vi "Sample Request Control.vi"(0 "Sample Request":bool, 2 "DOUTs OFF":bool, 4 "SimDINs":bool[](array[boolean])=[FALSE, FALSE, FALSE, FALSE, FALSE], 5 "ErrIn":errorcluster, 6 "PC ID":i32=1, 7 "SimOn":bool, 8 "PC1 In Inv":bool[](array[boolean])=[FALSE, FALSE, FALSE, FALSE, FALSE], 9 "Init":bool, 10 "Lockout Inv":bool, 11 "Reset":bool, 13 "Stop":bool) -> (14 "Request Granted":bool, 15 "Lockout Status":bool, 16 "Reset Done":bool, 17 "State":T1(ring), 18 "Busy Status":bool[](array[boolean]), 19 "ErrOut":errorcluster)   [LabVIEW 2013]
uses:
  <vilib>/DAQmx/write.llb/DAQmx Write (Digital Bool 1Line 1Point).vi
  <vilib>/DAQmx/read.llb/DAQmx Read (Digital 1D Bool NChan 1Samp 1Line).vi
  <vilib>/DAQmx/miscellaneous.llb/DAQmx Fill In Error Info.vi
  <vilib>/DAQmx/create/channels.llb/DAQmx Create Channel (DI-Digital Input).vi
  <vilib>/DAQmx/create/channels.llb/DAQmx Create Channel (DO-Digital Output).vi
panel:
  in  "PC1 In Line Grouping":i32(ring) items=["one channel for each line", "one channel for all lines"]
  in  "PC1 In Chls":tag="Dev1/port2/line0:1"
  in  "PC1 Out Line Grouping":i32(ring) items=["one channel for each line", "one channel for all lines"]
  in  "PC1 Out Chls":tag="Dev1/port1/line6"
  # "Input Parameters"
  # "ER2007"
  # "Output Parameters"
  # "Expected \"Sample Request\" Button Behavior:\n(1) A transition from FALSE to TRUE signals the start of a new\n     request.  If the other PC is not in the middle of a sample,\n     this vi sets \"Request Granted\" to TRUE and asserts the\n     \"Lockout\" line.  On the next loop iteration, \"Sample Request\"\n     must be FALSE because global 'GCD Busy' is now TRUE.\n     This vi proceeds thru if phases and returns to the 'Idle' state,\n(2)  If the other PC was processing a sample (busy), then this vi\n      proceeds to the 'Check Again x' state.  So long as the \"Sample\n      Request\" remains TRUE, the Busy line is checked every loop\n      iteration until it is either FALSE or until the \"Reset\" button is\n      pushed.  If the Busy goes FALSE, the \"Request Granted\" and\n      the \"Lockout\" lines are asserted.\n(3)  An external \"Reset\" is required to return the \"Lockout\" line to\n      FALSE.  Output Boolean \"Lockout Done\" is pulsed high and\n      can be used to reset the Global variable used for resets.\n(4) The \"Request Granted\" Boolean is pulsed TRUE for one loop\n      iteration."
  # "PC #1 Input Channels"
  # "PC #1 Output Channel"
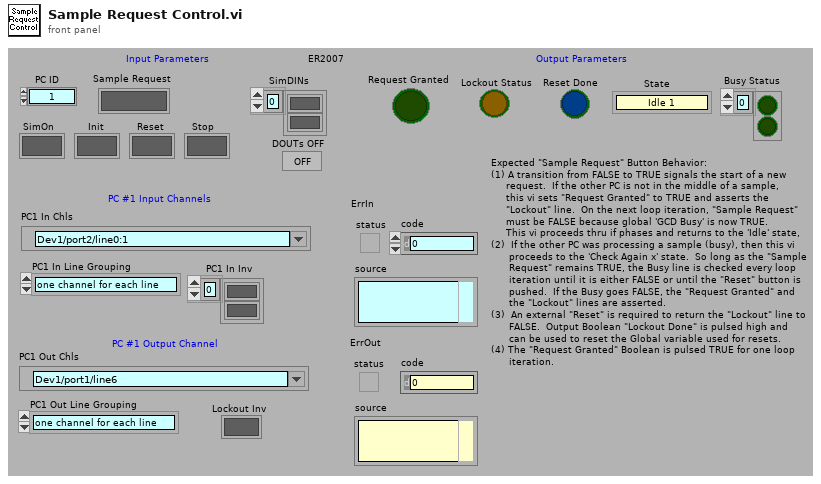
[diagram p1: front panel]
types:
  T1 = enum16{"Idle 1", "Request 1", "Check Again 1", "Done 1", "Idle 2", "Request 2", "Wait 2", "Check Again 2", "Done 2"}
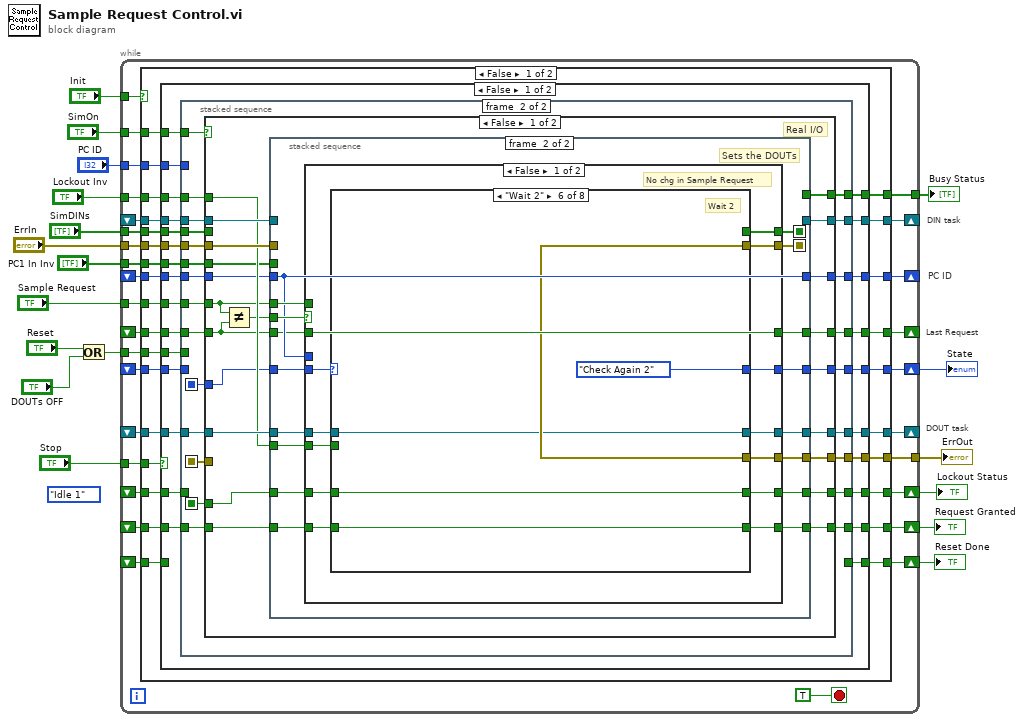
[diagram p0: block diagram]
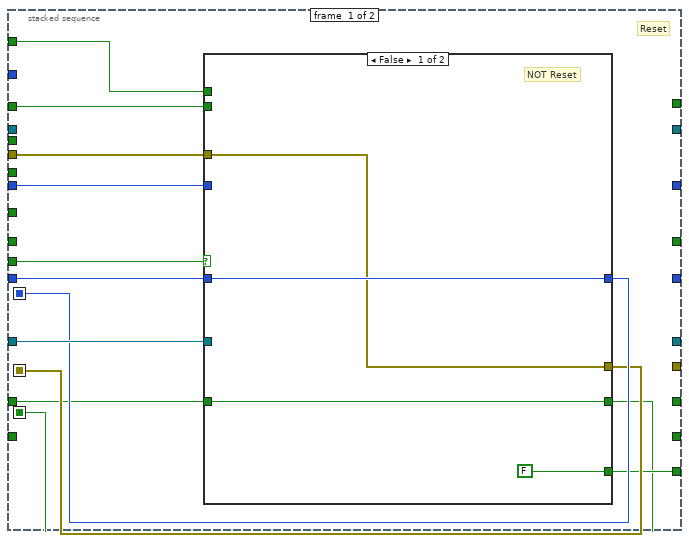
[diagram p2: hidden frame]
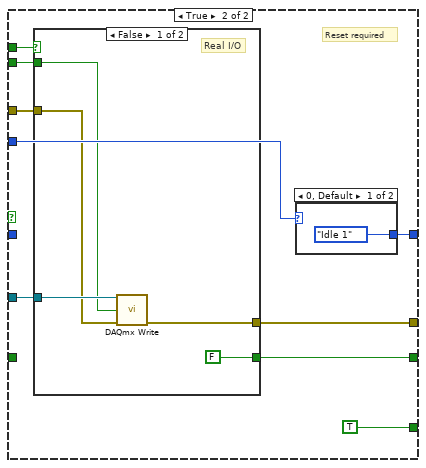
[diagram p3: hidden frame]
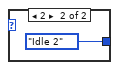
[diagram p4: hidden frame]
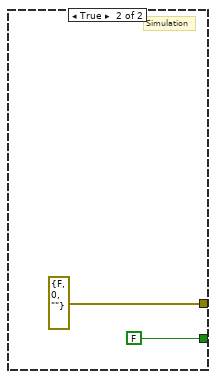
[diagram p5: hidden frame]
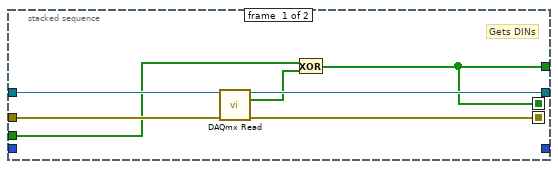
[diagram p6: hidden frame]
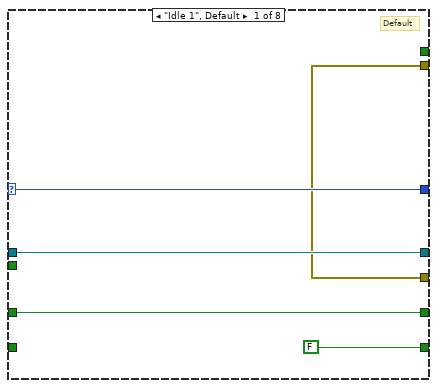
[diagram p7: hidden frame]
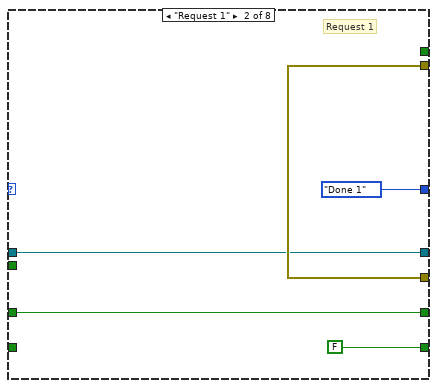
[diagram p8: hidden frame]
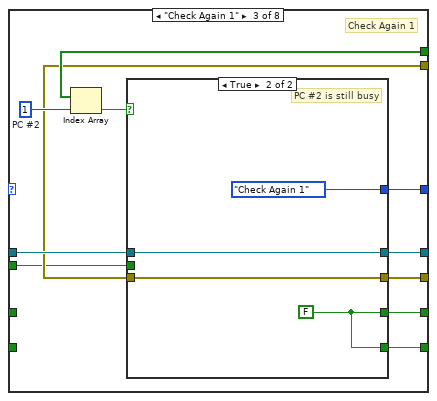
[diagram p9: hidden frame]
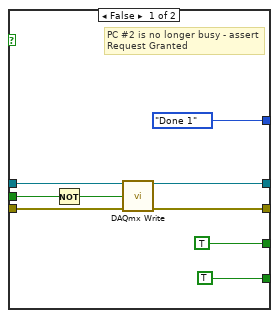
[diagram p10: hidden frame]
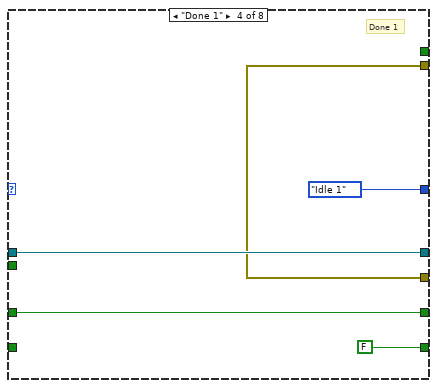
[diagram p11: hidden frame]
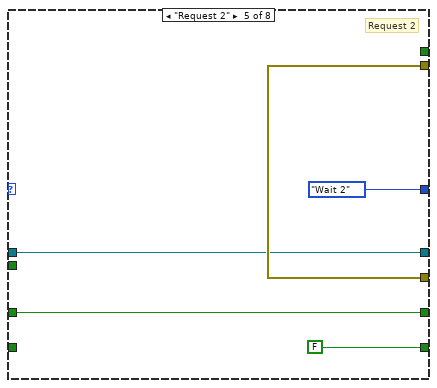
[diagram p12: hidden frame]
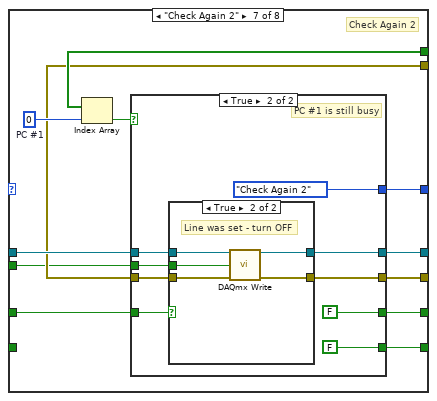
[diagram p13: hidden frame]
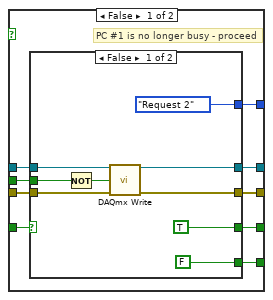
[diagram p14: hidden frame]
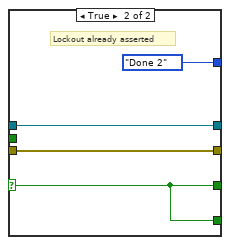
[diagram p15: hidden frame]
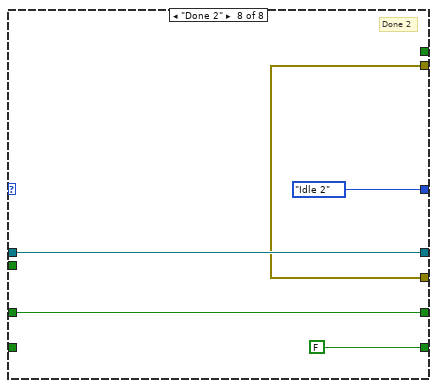
[diagram p17: hidden frame]
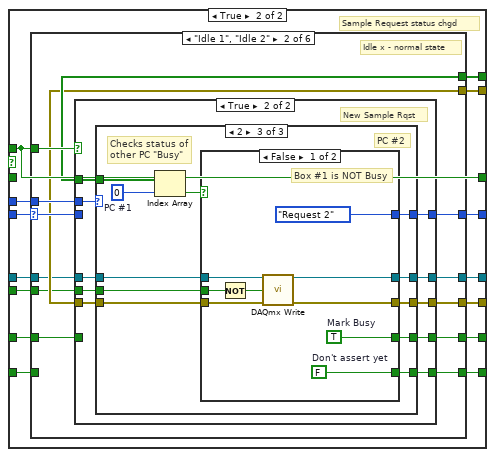
[diagram p18: hidden frame]
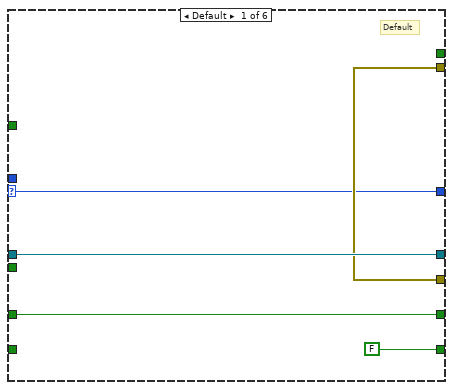
[diagram p19: hidden frame]
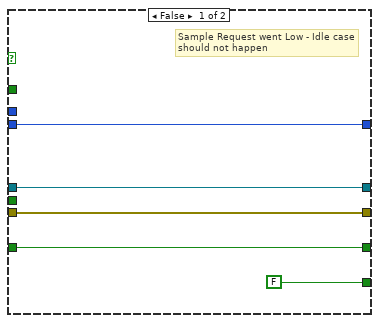
[diagram p20: hidden frame]
diagram:
  (unwired) T1."Idle 1"
  # "Last Request"
  # "DOUT task"
  # "DIN task"
  # "PC ID"
  n1 = Or(x="Reset", y="DOUTs OFF") -> (x .or. y?=w3:bool)
  n2 = while {
    tunnel: [w47] -> w8
    tunnel: "SimOn" -> [w46]
    tunnel: "Stop" -> [w44]
    shift-right: [w43] -> _
    shift-left: _ -> [w42]
    tunnel: "Init" -> [w40]
    tunnel: "PC ID" -> [w41]
    shift-right: [w39] -> _
    shift-left: _ -> [w37]
    tunnel: "Lockout Inv" -> [w38]
    tunnel: [w36] -> w14
    tunnel: "SimDINs" -> [w35]
    tunnel: "ErrIn" -> [w34]
    shift-right: [w33] -> _
    shift-left: _ -> [w32]
    tunnel: "Sample Request" -> [w31]
    shift-right: [w30] -> w10
    shift-left: _ -> [w27]
    shift-right: [w29] -> _
    shift-left: _ -> [w28]
    shift-right: [w26] -> w4
    shift-left: _ -> [w25]
    tunnel: w3 -> [w24]
    tunnel: "PC1 In Inv" -> [w23]
    shift-right: [w22] -> w7
    shift-left: _ -> [w21]
    shift-right: [w20] -> w6
    shift-left: _ -> [w19]
    stop <- TRUE stop-if-true
    n3 = case shown="False" w40 {
      tunnel: [w74 w676] -> w47
      tunnel: w46 -> [w73 w679]
      tunnel: w44 -> [w62 _]
      tunnel: [w72 w675] -> w43
      tunnel: w42 -> [w71 w669]
      tunnel: w41 -> [w50 w665]
      tunnel: [w68 w678] -> w39
      tunnel: w38 -> [w63 w677]
      tunnel: [w61 w674] -> w26
      tunnel: w37 -> [w69 w673]
      tunnel: w34 -> [w70 w672]
      tunnel: [w67 w671] -> w36
      tunnel: w35 -> [w66 w670]
      tunnel: [w60 w668] -> w33
      tunnel: w32 -> [w65 _]
      tunnel: w31 -> [w64 w667]
      tunnel: [w59 w666] -> w30
      tunnel: [w57 w665] -> w29
      tunnel: w28 -> [w58 _]
      tunnel: w27 -> [w56 _]
      tunnel: [w55 FALSE ("Sample Request")] -> w22
      tunnel: w25 -> [w54 _]
      tunnel: w24 -> [w53 _]
      tunnel: w23 -> [w52 _]
      tunnel: w21 -> [w51 _]
      tunnel: [w49 FALSE ("Don't assert yet")] -> w20
      tunnel: w19 -> [w48 _]
      frame False {
        n4 = case shown="False" w62 {
          tunnel: [w99 w648] -> w74
          tunnel: w73 -> [w98 w644]
          tunnel: [w97 refnum<k21> refnum ("task out")] -> w72
          tunnel: w71 -> [w96 w649]
          tunnel: w70 -> [w95 _]
          tunnel: w69 -> [w94 w652]
          tunnel: [w93 refnum<k21> refnum ("task out")] -> w68
          tunnel: [w92 bool[] [FALSE, FALSE]] -> w67
          tunnel: w66 -> [w91 _]
          tunnel: w65 -> [w80 _]
          tunnel: w64 -> [w81 _]
          tunnel: w63 -> [w90 w641]
          tunnel: [w84 w645] -> w61
          tunnel: [w87 FALSE] -> w60
          tunnel: [w86 w643] -> w59
          tunnel: w58 -> [w89 w642]
          tunnel: [w88 w642] -> w57
          tunnel: w56 -> [w85 _]
          tunnel: [w83 w645] -> w55
          tunnel: w54 -> [w82 _]
          tunnel: w53 -> [w78 _]
          tunnel: w52 -> [w75 _]
          tunnel: w51 -> [w79 _]
          tunnel: w50 -> [w77 _]
          tunnel: [w76 w645] -> w49
          tunnel: w48 -> [_ _]
          frame False {
            n5 = stacked-sequence {
              seq-local: [w102 _] -> [_ w135]
              seq-local: [w105 _] -> [_ w137]
              seq-local: [w104 _] -> [_ w136]
              tunnel: [_ w156] -> w99
              tunnel: w98 -> [w111 w155]
              tunnel: [_ w154] -> w97
              tunnel: w96 -> [w109 w153]
              tunnel: w95 -> [w108 w152]
              tunnel: w94 -> [_ w151]
              tunnel: [_ w150] -> w93
              tunnel: [_ w149] -> w92
              tunnel: w91 -> [_ w148]
              tunnel: w90 -> [w110 w147]
              tunnel: w89 -> [w101 w146]
              tunnel: [_ w145] -> w88
              tunnel: [_ w144] -> w87
              tunnel: [_ w143] -> w86
              tunnel: w85 -> [w106 _]
              tunnel: [_ w142] -> w84
              tunnel: [_ w141] -> w83
              tunnel: w82 -> [w100 _]
              tunnel: w81 -> [_ w140]
              tunnel: w80 -> [_ w139]
              tunnel: w79 -> [_ w138]
              tunnel: w78 -> [w107 _]
              tunnel: w77 -> [_ _]
              tunnel: [w103 _] -> w76
              tunnel: w75 -> [_ w134]
              frame #0 {
                # "Reset"
                n6 = case shown="False" w107 {
                  tunnel: w111 -> [_ w124]
                  tunnel: w110 -> [_ w123]
                  tunnel: w109 -> [_ w122]
                  tunnel: w108 -> [w114 w121]
                  tunnel: [w115 w117] -> w105
                  tunnel: w106 -> [w115 _]
                  tunnel: [w114 w120] -> w104
                  tunnel: [FALSE TRUE] -> w103
                  tunnel: [w112 w118] -> w102
                  tunnel: w101 -> [_ w116]
                  tunnel: w100 -> [w112 _]
                  frame False {
                    # "NOT Reset"
                  }
                  frame True {
                    # "Reset required"
                    n7 = case shown="False" w124 {
                      tunnel: w122 -> [w131 _]
                      tunnel: [FALSE FALSE] -> w118
                      tunnel: [w130 errorcluster {"status"=FALSE, "code"=0, "source"=""}] -> w120
                      tunnel: w123 -> [w129 _]
                      tunnel: w121 -> [w128 _]
                      frame False {
                        # "Real I/O"
                        n8 = call-poly <vilib>:"DAQmx Write.vi"("task/channels in"=w131, "data"=w129, "error in"=w128) -> ("error out"=w130:errorcluster)  [unwired: 10 in, 2 out]
                      }
                      frame True {
                        # "Simulation"
                      }
                    }
                    n9 = case shown="0, Default" w116 {
                      tunnel: [T1."Idle 1" T1."Idle 2"] -> w117
                      frame 0, Default {
                      }
                      frame 2 {
                      }
                    }
                  }
                }
              }
              frame #1 {
                n10 = case shown="False" w155 {
                  tunnel: [w177 w476] -> w156
                  tunnel: [w176 w477] -> w154
                  tunnel: w153 -> [w175 _]
                  tunnel: w146 -> [w169 w482]
                  tunnel: w152 -> [w174 _]
                  tunnel: w151 -> [w173 w467]
                  tunnel: [w172 w467] -> w150
                  tunnel: [w171 w483] -> w149
                  tunnel: w148 -> [_ w484]
                  tunnel: w140 -> [w166 w471]
                  tunnel: w139 -> [w157 w470]
                  tunnel: w147 -> [w170 _]
                  tunnel: [w159 w481] -> w145
                  tunnel: [w158 w480] -> w144
                  tunnel: [w164 w479] -> w143
                  tunnel: w137 -> [w163 w478]
                  tunnel: [w168 w475] -> w142
                  tunnel: [w167 w474] -> w141
                  tunnel: w135 -> [w162 w473]
                  tunnel: w138 -> [w161 w469]
                  tunnel: w136 -> [_ w468]
                  tunnel: w134 -> [w160 _]
                  frame False {
                    # "Real I/O"
                    n11 = Not Equal?(x=w166, y=w157) -> (x != y?=w165:bool)
                    n12 = stacked-sequence {
                      seq-local: [w182 _] -> [_ w198]
                      seq-local: [w179 _] -> [_ w190]
                      tunnel: [_ w201] -> w177
                      tunnel: [_ w200] -> w176
                      tunnel: w175 -> [_ w199]
                      tunnel: w169 -> [_ w187]
                      tunnel: w174 -> [w184 _]
                      tunnel: w173 -> [w183 _]
                      tunnel: [w181 _] -> w172
                      tunnel: [w179 _] -> w171
                      tunnel: w170 -> [_ w188]
                      tunnel: [_ w197] -> w168
                      tunnel: [_ w196] -> w167
                      tunnel: w166 -> [_ w195]
                      tunnel: w165 -> [_ w194]
                      tunnel: [_ w193] -> w164
                      tunnel: w163 -> [_ w192]
                      tunnel: w162 -> [_ w191]
                      tunnel: w161 -> [_ w189]
                      tunnel: w160 -> [w178 _]
                      tunnel: [_ w187] -> w159
                      tunnel: [_ w186] -> w158
                      tunnel: w157 -> [_ w185]
                      frame #0 {
                        # "Gets DINs"
                        n13 = call-poly <vilib>:"DAQmx Read.vi"("task/channels in"=w183, "error in"=w184) -> ("task out"=w181:refnum<k21>, "data"=w180:bool[], "error out"=w182:errorcluster)  [unwired: 11 in]
                        n14 = Exclusive Or(1:w180, 2:w178) -> (0:w179:bool[])
                      }
                      frame #1 {
                        # "Sets the DOUTs"
                        n15 = case shown="False" w194 {
                          tunnel: [w209 w332] -> w201
                          tunnel: [w211 w331] -> w200
                          tunnel: w199 -> [w212 w330]
                          tunnel: w187 -> [_ w323]
                          tunnel: w188 -> [w204 w321]
                          tunnel: w198 -> [w210 w329]
                          tunnel: [w207 w328] -> w197
                          tunnel: [w208 w327] -> w196
                          tunnel: w195 -> [_ w319]
                          tunnel: [w214 w324] -> w193
                          tunnel: w192 -> [w213 w326]
                          tunnel: w191 -> [w206 w325]
                          tunnel: w190 -> [w205 w322]
                          tunnel: w189 -> [w203 w320]
                          tunnel: [w202 w319] -> w186
                          tunnel: w185 -> [w202 _]
                          frame False {
                            # "No chg in Sample Request"
                            n16 = case shown="\"Wait 2\"" w213 {
                              selector: w213 -> [w219 _ _ _ _ _ _ _]
                              tunnel: [w219 T1."Done 1" w232 T1."Idle 1" T1."Wait 2" T1."Check Again 2" w272 T1."Idle 2"] -> w214
                              tunnel: w212 -> [w218 w223 w231 w252 w256 w261 w266 w316]
                              tunnel: [w218 w223 w228 w252 w256 w261 w267 w316] -> w211
                              tunnel: w210 -> [w217 w224 w229 w251 w257 w262 w265 w315]
                              tunnel: [w217 w224 w227 w251 w257 w262 w268 w315] -> w209
                              tunnel: [FALSE FALSE w230 FALSE FALSE w260 w269 FALSE ("Don't assert yet")] -> w208
                              tunnel: [w215 w222 w225 w250 w255 w259 w270 w314] -> w207
                              tunnel: w206 -> [w215 w222 _ w250 w255 w259 w271 w314]
                              tunnel: w205 -> [_ _ w235 _ _ _ w273 _]
                              tunnel: w204 -> [_ _ w226 _ _ _ w264 _]
                              tunnel: w203 -> [_ _ _ _ _ w260 _ _]
                              frame "Idle 1", Default {
                                # "Default"
                              }
                              frame "Request 1" {
                                # "Request 1"
                              }
                              frame "Check Again 1" {
                                w234 = 1  # PC #2
                                # "Check Again 1"
                                n17 = Index Array(array=w235, index=w234) -> (element=w233:bool)
                                n18 = case shown="True" w233 {
                                tunnel: [T1."Done 1" T1."Check Again 1"] -> w232
                                tunnel: w231 -> [w242 w247]
                                tunnel: [TRUE w245] -> w230
                                tunnel: w229 -> [w239 w246]
                                tunnel: [w241 w247] -> w228
                                tunnel: [w240 w246] -> w227
                                tunnel: w226 -> [w238 _]
                                tunnel: [TRUE w245] -> w225
                                frame False {
                                # "PC #2 is no longer busy - assert\nRequest Granted"
                                n19 = Not(x=w238) -> (.not. x?=w237:bool)
                                n20 = call-poly <vilib>:"DAQmx Write.vi"("task/channels in"=w242, "data"=w237, "error in"=w239) -> ("task out"=w241:refnum<k21>, "error out"=w240:errorcluster)  [unwired: 10 in, 1 out]
                                }
                                frame True {
                                w245 = FALSE
                                # "PC #2 is still busy"
                                }
                                }
                              }
                              frame "Done 1" {
                                # "Done 1"
                              }
                              frame "Request 2" {
                                # "Request 2"
                              }
                              frame "Wait 2" {
                                # "Wait 2"
                              }
                              frame "Check Again 2" {
                                w275 = 0  # PC #1
                                # "Check Again 2"
                                n21 = Index Array(array=w273, index=w275) -> (element=w274:bool)
                                n22 = case shown="True" w274 {
                                tunnel: [w282 T1."Check Again 2"] -> w272
                                tunnel: [w284 FALSE] -> w269
                                tunnel: [w283 FALSE] -> w270
                                tunnel: w271 -> [w281 w303]
                                tunnel: [w277 w300] -> w268
                                tunnel: [w279 w299] -> w267
                                tunnel: w266 -> [w280 w301]
                                tunnel: w265 -> [w278 w302]
                                tunnel: w264 -> [w276 w298]
                                frame False {
                                # "PC #1 is no longer busy - proceed"
                                n23 = case shown="False" w281 {
                                selector: w281 -> [_ w296]
                                tunnel: [FALSE w296] -> w284
                                tunnel: [TRUE w296] -> w283
                                tunnel: [T1."Request 2" T1."Done 2"] -> w282
                                tunnel: w280 -> [w290 w294]
                                tunnel: [w289 w294] -> w279
                                tunnel: w278 -> [w288 w295]
                                tunnel: [w287 w295] -> w277
                                tunnel: w276 -> [w286 _]
                                frame False {
                                n24 = Not(x=w286) -> (.not. x?=w285:bool)
                                n25 = call-poly <vilib>:"DAQmx Write.vi"("task/channels in"=w290, "data"=w285, "error in"=w288) -> ("task out"=w289:refnum<k21>, "error out"=w287:errorcluster)  [unwired: 10 in, 1 out]
                                }
                                frame True {
                                # "Lockout already asserted"
                                }
                                }
                                }
                                frame True {
                                # "PC #1 is still busy"
                                n26 = case shown="True" w303 {
                                tunnel: w302 -> [w307 w310]
                                tunnel: w301 -> [w308 w313]
                                tunnel: [w307 w311] -> w300
                                tunnel: [w308 w312] -> w299
                                tunnel: w298 -> [_ w309]
                                frame False {
                                }
                                frame True {
                                # "Line was set - turn OFF"
                                n27 = call-poly <vilib>:"DAQmx Write.vi"("task/channels in"=w313, "data"=w309, "error in"=w310) -> ("task out"=w312:refnum<k21>, "error out"=w311:errorcluster)  [unwired: 10 in, 1 out]
                                }
                                }
                                }
                                }
                              }
                              frame "Done 2" {
                                # "Done 2"
                              }
                            }
                          }
                          frame True {
                            # "Sample Request status chgd"
                            n28 = case shown="\"Idle 1\", \"Idle 2\"" w326 {
                              selector: w326 -> [w333 w345 _ _ w438 _]
                              tunnel: [w336 w342 w421 w426 w434 w460] -> w332
                              tunnel: [w337 w340 w423 w427 w435 w462] -> w331
                              tunnel: w330 -> [w337 w339 w423 w427 w433 w462]
                              tunnel: w329 -> [w336 w341 w421 w426 w432 w460]
                              tunnel: [w334 w350 w422 w428 w442 w461] -> w328
                              tunnel: [FALSE w349 FALSE FALSE w441 FALSE ("Don't assert yet")] -> w327
                              tunnel: w325 -> [w334 w343 w422 w428 w437 w461]
                              tunnel: [w333 w348 T1."Done 1" T1."Wait 2" w443 w464] -> w324
                              tunnel: w323 -> [_ w347 _ _ w439 w463]
                              tunnel: w319 -> [_ w346 _ _ w440 _]
                              tunnel: w322 -> [_ w344 _ _ _ _]
                              tunnel: w321 -> [_ w338 _ _ w431 _]
                              tunnel: w320 -> [_ _ _ _ w436 _]
                              frame Default {
                                # "Default"
                              }
                              frame "Idle 1", "Idle 2" {
                                # "Idle x - normal state"
                                n29 = case shown="True" w346 {
                                tunnel: [w355 w365] -> w348
                                tunnel: w347 -> [_ w364]
                                tunnel: w345 -> [w355 _]
                                tunnel: w344 -> [_ w363]
                                tunnel: [FALSE w362] -> w349
                                tunnel: [w353 w361] -> w350
                                tunnel: w343 -> [w353 _]
                                tunnel: [w352 w359] -> w342
                                tunnel: w341 -> [w352 w357]
                                tunnel: [w351 w360] -> w340
                                tunnel: w339 -> [w351 w358]
                                tunnel: w338 -> [_ w356]
                                frame False {
                                # "Sample Request went Low - Idle case\nshould not happen"
                                }
                                frame True {
                                # "New Sample Rqst"
                                n30 = case shown="2" w364 {
                                tunnel: [T1."Idle 1" w378 w403] -> w365
                                tunnel: w363 -> [_ w381 w406]
                                tunnel: [FALSE w377 w402] -> w362
                                tunnel: [FALSE w376 w401] -> w361
                                tunnel: [w367 w375 w397] -> w360
                                tunnel: [w366 w374 w398] -> w359
                                tunnel: w358 -> [w367 w373 w400]
                                tunnel: w357 -> [w366 w372 w399]
                                tunnel: w356 -> [_ w371 w396]
                                frame 0, Default {
                                # "Invalid PC # - should never happen"
                                }
                                frame 1 {
                                w380 = 1  # PC #2
                                # "Checks status of\nother PC \"Busy\""
                                # "PC #1"
                                n31 = Index Array(array=w381, index=w380) -> (element=w379:bool)
                                n32 = case shown="True" w379 {
                                tunnel: [T1."Request 1" T1."Check Again 1"] -> w378
                                tunnel: [TRUE FALSE] -> w377
                                tunnel: [TRUE FALSE] -> w376
                                tunnel: [w386 w392] -> w375
                                tunnel: [w385 w391] -> w374
                                tunnel: w373 -> [w387 w392]
                                tunnel: w372 -> [w384 w391]
                                tunnel: w371 -> [w383 _]
                                frame False {
                                # "Box #2 is NOT Busy"
                                n33 = Not(x=w383) -> (.not. x?=w382:bool)
                                n34 = call-poly <vilib>:"DAQmx Write.vi"("task/channels in"=w387, "data"=w382, "error in"=w384) -> ("task out"=w386:refnum<k21>, "error out"=w385:errorcluster)  [unwired: 10 in, 1 out]
                                }
                                frame True {
                                # "Box #2 is Busy"
                                }
                                }
                                }
                                frame 2 {
                                w405 = 0  # PC #1
                                # "Checks status of\nother PC \"Busy\""
                                # "PC #2"
                                n35 = Index Array(array=w406, index=w405) -> (element=w404:bool)
                                n36 = case shown="False" w404 {
                                tunnel: [T1."Request 2" T1."Check Again 2"] -> w403
                                tunnel: [w415 FALSE] -> w402
                                tunnel: [w414 FALSE] -> w401
                                tunnel: w400 -> [w412 w417]
                                tunnel: w399 -> [w411 w416]
                                tunnel: [w409 w416] -> w398
                                tunnel: [w410 w417] -> w397
                                tunnel: w396 -> [w408 _]
                                frame False {
                                w414 = TRUE  # Mark Busy
                                w415 = FALSE  # Don't assert yet
                                # "Box #1 is NOT Busy"
                                n37 = Not(x=w408) -> (.not. x?=w407:bool)
                                n38 = call-poly <vilib>:"DAQmx Write.vi"("task/channels in"=w412, "data"=w407, "error in"=w411) -> ("task out"=w410:refnum<k21>, "error out"=w409:errorcluster)  [unwired: 10 in, 1 out]
                                }
                                frame True {
                                # "Box #1 is Busy"
                                }
                                }
                                }
                                }
                                }
                                }
                              }
                              frame "Request 1" {
                                # "Request 1"
                              }
                              frame "Request 2" {
                                # "Request 2"
                              }
                              frame "Check Again 1", "Check Again 2" {
                                # "Check Again x"
                                n39 = case shown="False" w440 {
                                tunnel: w436 -> [_ w457]
                                tunnel: w437 -> [_ w458]
                                tunnel: [w449 w458] -> w442
                                tunnel: [w449 w457] -> w441
                                tunnel: w438 -> [_ w456]
                                tunnel: [w451 w456] -> w443
                                tunnel: w439 -> [w450 _]
                                tunnel: [w447 w455] -> w435
                                tunnel: [w445 w454] -> w434
                                tunnel: w433 -> [w448 w455]
                                tunnel: w432 -> [w446 w454]
                                tunnel: w431 -> [w444 _]
                                frame False {
                                w449 = FALSE
                                # "Resets to Idle"
                                n40 = case shown="1, Default" w450 {
                                tunnel: [T1."Idle 1" T1."Idle 2"] -> w451
                                frame 1, Default {
                                }
                                frame 2 {
                                }
                                }
                                n41 = call-poly <vilib>:"DAQmx Write.vi"("task/channels in"=w448, "data"=w444, "error in"=w446) -> ("task out"=w447:refnum<k21>, "error out"=w445:errorcluster)  [unwired: 10 in, 1 out]
                                }
                                frame True {
                                }
                                }
                              }
                              frame "Done 1", "Done 2" {
                                # "Done x"
                                n42 = case shown="1, Default" w463 {
                                tunnel: [T1."Idle 1" T1."Idle 2"] -> w464
                                frame 1, Default {
                                }
                                frame 2 {
                                }
                                }
                              }
                            }
                          }
                        }
                      }
                    }
                  }
                  frame True {
                    # "Simulation"
                    n43 = Not Equal?(x=w471, y=w470) -> (x != y?=w472:bool)
                    n44 = stacked-sequence {
                      seq-local: [w486 _] -> [_ w492]
                      seq-local: [w485 _] -> [_ w494]
                      tunnel: w484 -> [w486 _]
                      tunnel: [w486 _] -> w483
                      tunnel: w472 -> [_ w500]
                      tunnel: w482 -> [_ w496]
                      tunnel: [_ w496] -> w481
                      tunnel: [_ w499] -> w480
                      tunnel: w471 -> [_ w487]
                      tunnel: [_ w498] -> w479
                      tunnel: w478 -> [_ w497]
                      tunnel: [_ refnum<k21> refnum ("task out")] -> w477
                      tunnel: [_ w494] -> w476
                      tunnel: [_ w493] -> w475
                      tunnel: [_ w491] -> w474
                      tunnel: w473 -> [_ w490]
                      tunnel: w470 -> [_ w489]
                      tunnel: w469 -> [_ w488]
                      tunnel: w468 -> [w485 _]
                      frame #0 {
                        # "Sims DINs"
                      }
                      frame #1 {
                        # "Sim DOUTs"
                        n45 = case shown="True" w500 {
                          tunnel: [w508 w565] -> w499
                          tunnel: w487 -> [_ w565]
                          tunnel: [w506 w566] -> w498
                          tunnel: w497 -> [w507 w564]
                          tunnel: w496 -> [_ w563]
                          tunnel: [w502 w560] -> w493
                          tunnel: w492 -> [w503 w562]
                          tunnel: [w504 w561] -> w491
                          tunnel: w490 -> [w501 w559]
                          tunnel: w489 -> [w508 _]
                          tunnel: w488 -> [w505 w558]
                          frame False {
                            # "No chg in Sample Request"
                            n46 = case shown="\"Idle 1\", Default" w507 {
                              selector: w507 -> [w511 _ _ _ _ _ _ _]
                              tunnel: [w511 T1."Done 1" w520 T1."Idle 1" T1."Wait 2" T1."Check Again 2" w541 T1."Idle 2"] -> w506
                              tunnel: w505 -> [_ _ _ _ w532 w535 _ _]
                              tunnel: [FALSE ("Don't assert yet") FALSE ("Don't assert yet") w518 FALSE ("Don't assert yet") w532 w535 w540 FALSE ("Don't assert yet")] -> w504
                              tunnel: w503 -> [_ _ w517 _ _ _ w542 _]
                              tunnel: [w509 w513 w519 w529 w531 w534 w539 w557] -> w502
                              tunnel: w501 -> [w509 w513 _ w529 w531 w534 w538 w557]
                              frame "Idle 1", Default {
                                # "Default"
                              }
                              frame "Request 1" {
                                # "Request 1"
                              }
                              frame "Check Again 1" {
                                w516 = 1  # PC #2
                                # "Check Again 1"
                                n47 = Index Array(array=w517, index=w516) -> (element=w515:bool)
                                n48 = case shown="True" w515 {
                                tunnel: [T1."Done 1" T1."Check Again 1"] -> w520
                                tunnel: [TRUE FALSE] -> w518
                                tunnel: [TRUE FALSE] -> w519
                                frame False {
                                # "PC #2 is no longer busy - assert\nRequest Granted"
                                }
                                frame True {
                                # "PC #2 is still busy"
                                }
                                }
                              }
                              frame "Done 1" {
                                # "Done 1"
                              }
                              frame "Request 2" {
                                # "Request 2"
                              }
                              frame "Wait 2" {
                                # "Wait 2"
                              }
                              frame "Check Again 2" {
                                w537 = 0  # PC #1
                                # "Check Again 2"
                                n49 = Index Array(array=w542, index=w537) -> (element=w536:bool)
                                n50 = case shown="False" w536 {
                                tunnel: [w544 T1."Check Again 2"] -> w541
                                tunnel: [w546 FALSE] -> w540
                                tunnel: [w545 FALSE] -> w539
                                tunnel: w538 -> [w543 _]
                                frame False {
                                # "PC #1 is no longer busy - proceed"
                                n51 = case shown="False" w543 {
                                selector: w543 -> [_ w550]
                                tunnel: [FALSE w550] -> w546
                                tunnel: [TRUE w550] -> w545
                                tunnel: [T1."Request 2" T1."Done 2"] -> w544
                                frame False {
                                }
                                frame True {
                                # "Lockout already asserted"
                                }
                                }
                                }
                                frame True {
                                # "PC #1 is still busy"
                                }
                                }
                              }
                              frame "Done 2" {
                                # "Done 2"
                              }
                            }
                          }
                          frame True {
                            # "Sample Request status chgd"
                            n52 = case shown="Default" w564 {
                              selector: w564 -> [w569 w574 _ _ w621 _]
                              tunnel: [w569 w577 T1."Done 1" T1."Wait 2" w620 w638] -> w566
                              tunnel: w565 -> [_ w576 _ _ w626 _]
                              tunnel: w563 -> [_ w575 _ _ w619 w635]
                              tunnel: w562 -> [_ w573 _ _ _ _]
                              tunnel: [FALSE ("Don't assert yet") w572 FALSE FALSE w622 FALSE ("Don't assert yet")] -> w561
                              tunnel: [w568 w571 w615 w618 w623 w637] -> w560
                              tunnel: w559 -> [w568 w570 w615 w618 w624 w637]
                              tunnel: w558 -> [_ _ _ _ w625 _]
                              frame Default {
                                # "Default"
                              }
                              frame "Idle 1", "Idle 2" {
                                # "Idle x - normal state"
                                n53 = case shown="True" w576 {
                                tunnel: [w580 w585] -> w577
                                tunnel: w575 -> [_ w584]
                                tunnel: w574 -> [w580 _]
                                tunnel: w573 -> [_ w583]
                                tunnel: [FALSE w582] -> w572
                                tunnel: [w578 w581] -> w571
                                tunnel: w570 -> [w578 _]
                                frame False {
                                # "Sample Request went Low - Idle case\nshould not happen"
                                }
                                frame True {
                                # "New Sample Rqst"
                                n54 = case shown="0, Default" w584 {
                                tunnel: [T1."Idle 1" w591 w603] -> w585
                                tunnel: w583 -> [_ w594 w606]
                                tunnel: [FALSE w590 w602] -> w582
                                tunnel: [FALSE w589 w601] -> w581
                                frame 0, Default {
                                # "Invalid PC # - should never happen"
                                }
                                frame 1 {
                                w593 = 1  # PC #2
                                # "Checks status of\nother PC \"Busy\""
                                # "PC #1"
                                n55 = Index Array(array=w594, index=w593) -> (element=w592:bool)
                                n56 = case shown="True" w592 {
                                tunnel: [T1."Request 1" T1."Check Again 1"] -> w591
                                tunnel: [TRUE FALSE] -> w590
                                tunnel: [TRUE FALSE] -> w589
                                frame False {
                                # "Box #2 is NOT Busy"
                                }
                                frame True {
                                # "Box #2 is Busy"
                                }
                                }
                                }
                                frame 2 {
                                w605 = 0  # PC #1
                                # "Checks status of\nother PC \"Busy\""
                                # "PC #2"
                                n57 = Index Array(array=w606, index=w605) -> (element=w604:bool)
                                n58 = case shown="True" w604 {
                                tunnel: [T1."Request 2" T1."Check Again 2"] -> w603
                                tunnel: [w609 FALSE] -> w602
                                tunnel: [TRUE FALSE] -> w601
                                frame False {
                                w609 = FALSE  # Don't assert yet
                                # "Box #1 is NOT Busy"
                                }
                                frame True {
                                # "Box #1 is Busy"
                                }
                                }
                                }
                                }
                                }
                                }
                              }
                              frame "Request 1" {
                                # "Request 1"
                              }
                              frame "Request 2" {
                                # "Request 2"
                              }
                              frame "Check Again 1", "Check Again 2" {
                                # "Check Again x"
                                n59 = case shown="False" w626 {
                                tunnel: w625 -> [_ w633]
                                tunnel: w624 -> [_ w634]
                                tunnel: [w627 w634] -> w623
                                tunnel: [w627 w633] -> w622
                                tunnel: w621 -> [_ w632]
                                tunnel: [w629 w632] -> w620
                                tunnel: w619 -> [w628 _]
                                frame False {
                                w627 = FALSE
                                # "Resets to Idle"
                                n60 = case shown="1, Default" w628 {
                                tunnel: [T1."Idle 1" T1."Idle 2"] -> w629
                                frame 1, Default {
                                }
                                frame 2 {
                                }
                                }
                                }
                                frame True {
                                }
                                }
                              }
                              frame "Done 1", "Done 2" {
                                # "Done x"
                                n61 = case shown="1, Default" w635 {
                                tunnel: [T1."Idle 1" T1."Idle 2"] -> w638
                                frame 1, Default {
                                }
                                frame 2 {
                                }
                                }
                              }
                            }
                          }
                        }
                      }
                    }
                  }
                }
              }
            }
          }
          frame True {
            w645 = FALSE
            # "Stop"
            n62 = case shown="True" w644 {
              tunnel: w652 -> [w661 _]
              tunnel: w649 -> [w657 _]
              tunnel: [w660 errorcluster {"status"=FALSE, "code"=0, "source"=""} ("error out")] -> w648
              tunnel: w641 -> [w655 _]
              frame False {
                # "Real I/O - clears tasks\nand resets Lockout"
                n63 = call <vilib>:"DAQmx Clear Task.vi"("task in"=w661) -> ("error out"=w658:errorcluster)  [unwired: 14 in]
                n64 = call-poly <vilib>:"DAQmx Write.vi"("task/channels in"=w657, "data"=w655, "error in"=w658) -> ("task out"=w656:refnum<k21>, "error out"=w659:errorcluster)  [unwired: 10 in, 1 out]
                n65 = call <vilib>:"DAQmx Clear Task.vi"("task in"=w656, "error in"=w659) -> ("error out"=w660:errorcluster)  [unwired: 13 in]
              }
              frame True {
                # "Sim"
              }
            }
            n66 = case shown="0, Default" w642 {
              tunnel: [T1."Idle 1" T1."Idle 2"] -> w643
              frame 0, Default {
              }
              frame 2 {
              }
            }
          }
        }
      }
      frame True {
        # "Init"
        n67 = case shown="False" w679 {
          tunnel: w665 -> [w693 _]
          tunnel: [w692 w744] -> w678
          tunnel: w677 -> [w691 _]
          tunnel: [w690 w742] -> w676
          tunnel: [w689 w741] -> w675
          tunnel: [w688 w740] -> w674
          tunnel: w673 -> [w687 _]
          tunnel: w672 -> [w686 _]
          tunnel: [w685 w745] -> w671
          tunnel: w670 -> [_ w743]
          tunnel: w669 -> [w684 _]
          tunnel: [w683 w739] -> w668
          tunnel: w667 -> [w682 _]
          frame False {
            # "Real I/O"
            n68 = stacked-sequence {
              seq-local: [w694 _] -> [_ w715]
              tunnel: w693 -> [w698 w721]
              tunnel: [w699 _] -> w692
              tunnel: w691 -> [_ w720]
              tunnel: [_ w719] -> w690
              tunnel: [_ w718] -> w689
              tunnel: [_ w717] -> w688
              tunnel: w687 -> [w697 _]
              tunnel: w686 -> [w696 _]
              tunnel: [w695 _] -> w685
              tunnel: w684 -> [_ w716]
              tunnel: [_ w714] -> w683
              tunnel: w682 -> [_ w713]
              frame #0 {
                # "DINs"
                n69 = case shown="0, Default" w698 {
                  tunnel: [w702 w709] -> w694
                  tunnel: [refnum<k21> refnum ("task out") w707] -> w699
                  tunnel: w697 -> [_ _]
                  tunnel: w696 -> [w702 w703]
                  tunnel: [bool[] [FALSE, FALSE] ("data") w704] -> w695
                  frame 0, Default {
                    # "Undefined PC #"
                  }
                  frame 1, 2 {
                    # "PC #'s 1 & 2"
                    n70 = call-poly <vilib>:"DAQmx Create Virtual Channel.vi"("lines"="PC1 In Chls", "line grouping"="PC1 In Line Grouping", "error in"=w703) -> ("task out"=w711:refnum<k21>, "error out"=w712:errorcluster)  [unwired: 11 in]
                    n71 = call <vilib>:"DAQmx Start Task.vi"("task/channels in"=w711, "error in"=w712) -> ("task out"=w708:refnum<k21>, "error out"=w710:errorcluster)  [unwired: 12 in]
                    n72 = call-poly <vilib>:"DAQmx Read.vi"("task/channels in"=w708, "error in"=w710) -> ("task out"=w707:refnum<k21>, "data"=w704:bool[], "error out"=w709:errorcluster)  [unwired: 11 in]
                  }
                }
              }
              frame #1 {
                # "DOUTs"
                n73 = case shown="1, 2" w721 {
                  tunnel: [w724 w731] -> w719
                  tunnel: [refnum<k21> refnum ("task out") w730] -> w718
                  tunnel: w720 -> [_ w729]
                  tunnel: [FALSE FALSE] -> w717
                  tunnel: w716 -> [_ _]
                  tunnel: w715 -> [w724 w728]
                  tunnel: [FALSE FALSE] -> w714
                  tunnel: w713 -> [_ _]
                  frame 0, Default {
                    # "Undefined PC #"
                  }
                  frame 1, 2 {
                    # "PC #'s 1 & 2"
                    n74 = call-poly <vilib>:"DAQmx Create Virtual Channel.vi"("lines"="PC1 Out Chls", "line grouping"="PC1 Out Line Grouping", "error in"=w728) -> ("task out"=w732:refnum<k21>, "error out"=w733:errorcluster)  [unwired: 11 in]
                    n75 = call <vilib>:"DAQmx Start Task.vi"("task/channels in"=w732, "error in"=w733) -> ("task out"=w737:refnum<k21>, "error out"=w738:errorcluster)  [unwired: 12 in]
                    n76 = call-poly <vilib>:"DAQmx Write.vi"("task/channels in"=w737, "auto start"=FALSE, "data"=w729, "error in"=w738) -> ("task out"=w730:refnum<k21>, "error out"=w731:errorcluster)  [unwired: 9 in, 1 out]
                  }
                }
              }
            }
          }
          frame True {
            # "Simulation"
            n77 = stacked-sequence {
              seq-local: [w747 _] -> [_ _]
              seq-local: [errorcluster {"status"=FALSE, "code"=0, "source"=""} ("error out") _] -> [_ w751]
              tunnel: [w747 _] -> w745
              tunnel: [refnum<k21> refnum ("task out") _] -> w744
              tunnel: w743 -> [w747 _]
              tunnel: [_ w751] -> w742
              tunnel: [_ refnum<k21> refnum ("task out")] -> w741
              tunnel: [_ FALSE] -> w740
              tunnel: [_ FALSE] -> w739
              frame #0 {
                # "DINs"
              }
              frame #1 {
                # "DOUTs"
              }
            }
          }
        }
        n78 = case shown="0, Default" w665 {
          tunnel: [T1."Idle 1" T1."Idle 2"] -> w666
          frame 0, Default {
          }
          frame 2 {
          }
        }
      }
    }
  }
  "ErrOut" <- w8
  "Request Granted" <- w7
  "Busy Status" <- w14
  "State" <- w10
  "Reset Done" <- w6
  "Lockout Status" <- w4
